vi "SavePatientDateInfo_Armpressure.vi"(8 "error in":errorcluster, 10 "Side(Left/Right)":string, 11 "Pressure":T1(array[cluster])) -> (0 "error out":errorcluster)   [LabVIEW 2013, in "main.lvlib"]
uses:
  main.lvlib
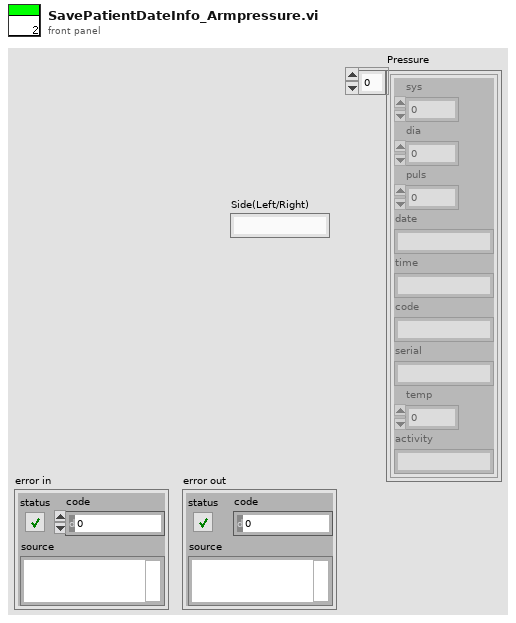
[diagram p1: front panel]
types:
  T1 = cluster{"sys":dbl, "dia":dbl, "puls":dbl, "date":string, "time":string, "code":string, "serial":string, "temp":dbl, "activity":string}[]
  T2 = typedef "main.lvlib/date_specific_info.ctl" = cluster{"profile":cluster{"id":string, "name":string, "operator":string, "doctor":string, "comment":string}, "hospital":cluster{"name":string, "department":string, "address":string}, "palpation":cluster{"right":string, "left":string}, "Armpressure Right":cluster{"sys":dbl, "dia":dbl, "puls":dbl, "date":string, "time":string, "code":string, "serial":string, "temp":dbl, "activity":string}[], "Armpressure Left":cluster{"sys":dbl, "dia":dbl, "puls":dbl, "date":string, "time":string, "code":string, "serial":string, "temp":dbl, "activity":string}[]}
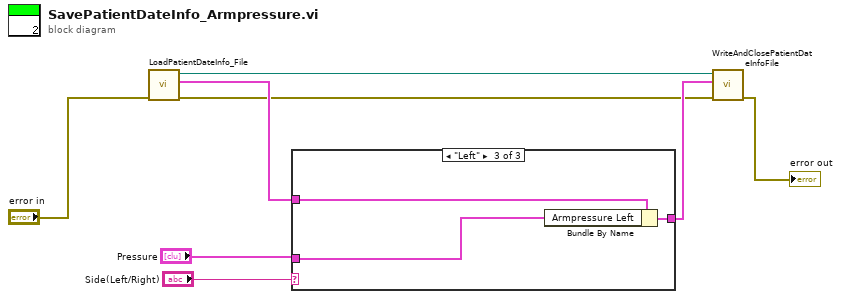
[diagram p0: block diagram]
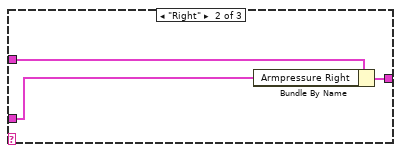
[diagram p3: hidden frame]
diagram:
  n1 = call "LoadPatientDateInfo_File.vi"("error in (no error)"="error in") -> ("error out"=w3:errorcluster, "date_specific_info"=w4:T2, "path"=w2:path)  [unwired: 8 in]
  n2 = case shown="\"Left\"" "Side(Left/Right)" {
    tunnel: [w9 w11 w15] -> w8
    tunnel: "Pressure" -> [_ w10 w13]
    tunnel: w4 -> [w9 w12 w14]
    frame "False", Default {
    }
    frame "Right" {
      n3 = Bundle By Name(cluster=w12, "Armpressure Right"=w10) -> (w11:T2)
    }
    frame "Left" {
      n4 = Bundle By Name(cluster=w14, "Armpressure Left"=w13) -> (w15:T2)
    }
  }
  n5 = call "WriteAndClosePatientDateInfoFile.vi"("error in (no error)"=w3, "date_specific_info"=w8, "file path (use dialog)"=w2) -> ("error out"=→"error out":errorcluster)  [unwired: 8 in]
